vi "AlliGator Find Python Function Information.vi"(8 "error in (no error)":errorcluster, 10 "Function Menu Item Tag":string, 11 "Target":string) -> (0 "error out":errorcluster, 3 "Python Function Info":T1={"Script Path"=path "", "Function Name"="", "Function Parent Menu"="", "Function Input Parameters"=[], "Function Outputs"=[], "Function Doc String"="", "Function Display Name"="", "Function Target Type"=enum."Window Menu", "Function Target Window"="", "Parent Menu Location"="", "Item Menu Tag"="", "Is preceded by Separator"=FALSE}, 4 "Found?":bool)   [LabVIEW 2021, in "AlliGator Python Plugins.lvlib"]
doc: "Gets python function's information."
uses:
  AlliGator Python Plugins.lvlib
  AlliGator Globals, Variables & Constants.lvlib
  AlliGator Variables List.ctl
  AlliGator Python Function Information.ctl
  AlliGator Python Function List.ctl
  <vilib>/ErrorRing/Error Ring.xnode
  AlliGator Python Function Parameter Definition.ctl
  AlliGator Python Plugin Target Type.ctl
  <vilib>/Utility/error.llb/Error Cluster From Error Code.vi
  AlliGator Python Function Output Definition.ctl
panel:
  # "see the AlliGator License on the block diagram (Ctrl+E or Window:Show Block Diagram)"
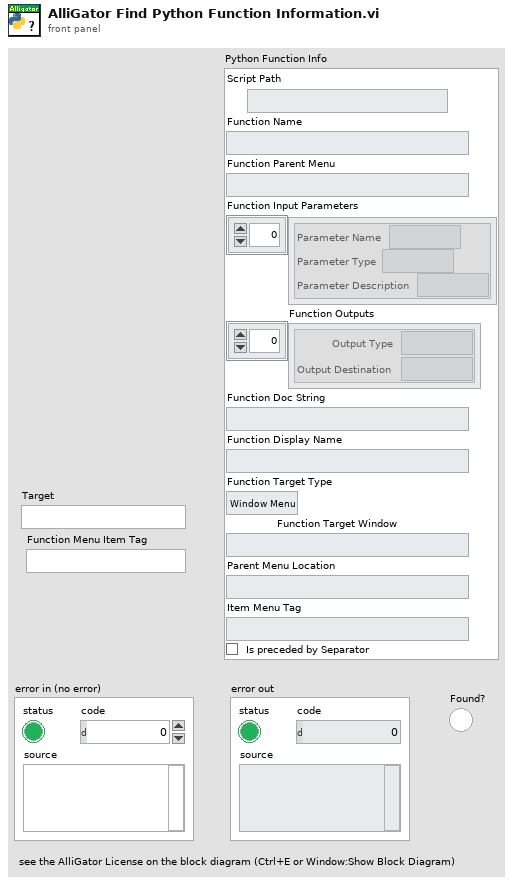
[diagram p1: front panel]
types:
  T1 = typedef "AlliGator Python Plugins.lvlib/AlliGator Python Function Information.ctl" = cluster{"Script Path":path, "Function Name":string, "Function Parent Menu":string, "Function Input Parameters":T2[], "Function Outputs":T3[], "Function Doc String":string, "Function Display Name":string, "Function Target Type":T4, "Function Target Window":string, "Parent Menu Location":string, "Item Menu Tag":string, "Is preceded by Separator":bool}
  T2 = typedef "AlliGator Python Plugins.lvlib/AlliGator Python Function Parameter Definition.ctl" = cluster{"Parameter Name":string, "Parameter Type":string, "Parameter Description":string}
  T3 = typedef "AlliGator Python Plugins.lvlib/AlliGator Python Function Output Definition.ctl" = cluster{"Output Type":string, "Output Destination":string}
  T4 = typedef "AlliGator Python Plugins.lvlib/AlliGator Python Plugin Target Type.ctl" = enum16{"Undefined", "Window Menu", "Object Menu"}
  T5 = typedef "AlliGator Python Plugins.lvlib/AlliGator Python Function List.ctl" = T1[]
  T6 = typedef "AlliGator Globals, Variables & Constants.lvlib/AlliGator Variables List.ctl" = enum16{"---- GUI ----", "GUI:Initialization Status", "GUI:State Indicators Refnum", "GUI:Original AlliGator Menu Items", "GUI:Current Action Loop State", "GUI:Script in progress", "GUI:Playback", "GUI:Loop Playback", "GUI:Search ROI Used", "GUI:Search ROI", "Decay Graph Max Legend Size", "Intensity Graph Max Legend Size", "Decay Statistics Graph Max Legend Size", "Phasor Graph Max Legend Size", "Phasor Ratio Graph Max Legend Size", "Lifetime Graph Max Legend Size", "---- Files ----", "Files:Export Dataset Frames as Individual Files", "Files:Show Batch Export Help Balloons", "Files:Frames in Dataset", "Files:ptu File Frame Start Indices", "Files:Current Frame in Dataset", "Files:Current Frame Timestamp", "Files:Dataset Loaded", "Files:Dataset Metadata", "Files:Dataset Channel", "Files:Dataset Data Description", "Files:Background Dataset Metadata", "Files:Background Dataset Channel", "Files:Background Dataset Data Description", "Files:Background File Subtraction", "Files:Background File Path", "Files:Background File Pile-up Correction", "Files:Background File Pixel Well Capacity", "Files:Background File Scaling Factor", "Files:Current Dataset Load Settings", "Files:Dataset Path", "------ Python Plugins ------", "Python Plugins:Information", "Python Plugins:Python Session", "Python Plugins:Valid Python Session?", "---- Source Image ----", "Source Image ROIs", "Current Source Image ROI", "Source Image ROI Event Refnum", "X_Source Image Display Range", "X_Source Image Palette Information", "Source Image Palette List", "Source Image Scale", "Source Image:ROI Overlay Color", "Source Image:ICCD-specific Information", "---- Image Profile Window ----", "Image Profile:Overlay ROI in Source Image", "Image Profile Window Event Refnum", "Image Profile:IntensityType", "Image Profile:Intensity Average Type", "Image Profile:Intensity-weighted SDV", "Image Profile:Box Profile Type", "Image Profile Window Open", "Image Profile:Plotted Fit Parameter", "X_Type of Displayed Image", "X_Time Gate Slider", "Source Image Overlay to Erase", "Is Displayed Image Accumulated", "White Light Image Modified", "Mask Image Modified", "Macrotime Gate Separation", "------ Phasor Graph -------", "Phasor Graph:Show Line", "---- Phasor Plot ---", "Phasor Plot Parameters Changed", "FLI Dataset Modified since last Phasor Plot Calculation", "Phasor Harmonics Data", "Selected Phasor Harmonics", "Phasor Harmonic Manager Event Refnum", "Phasor Plot ROIs", "Current Phasor Plot ROI", "Phasor Plot ROI Event Refnum", "Phasor Plot Image Reference Points", "Phasor Plot Computed", "Phasor Plot Palette Information", "Phasor Plot Palette List", "Phasor Ratio Palette Information", "Phasor Ratio Palette List", "Phasor Image Scale", "Phasor Plot Image Overlay to Erase", "Phasor Plot Image Elements to Update", "Current Phasor Plot Calculation Parameters", "Current Phasor Calibration Options", "Reset Cumulated Phasor Plot", "Phasor Ratio Reference 1", "Phasor Ratio Lifetime Reference 1", "Phasor Ratio Reference 1 Frequency", "Phasor Ratio Reference 2", "Phasor Ratio Lifetime Reference 2", "Phasor Ratio Reference 2 Frequency", "---- Decay Analysis ----", "Number of Selected Decays to Fit", "LS Fit Results", "LAR Fit Results", "BS Fit Results", "Last Decay Max - Min", "Best Fit Parameters", "Best Fit Parameter Names", "Actual Size X", "Actual Size Y", "Binning X", "Binning Y", "Actual # Gates", "Dataset Number", "Gates to...", "Gates Skipped", "Gates to keep", "Gate Step", "Gate Separation", "Reversed Gates", "Pile-up Correction", "Pixel Well Capacity", "Background Subtracted", "Background Subtraction Method", "Background Definition Range", "Background File (deprecated)", "Number of Dataset Accumulated", "Array of Accumulated Dataset Paths", "Do Averaged Datasets", "Destination File Path", "Process Plot Target", "Use 1/D as Phasor Frequency", "---- Decay Fit Parameter Map -----", "Decay Fit Parameter Map Palette Information", "Decay Fit Parameter Map Palette List", "Local Decay Graph Window Event Refnum", "------- Local Decay Window ---------", "Use normalized IRF for convolution", "----- Miscellaneous ----", "Skippable Dialog Windows Status"}
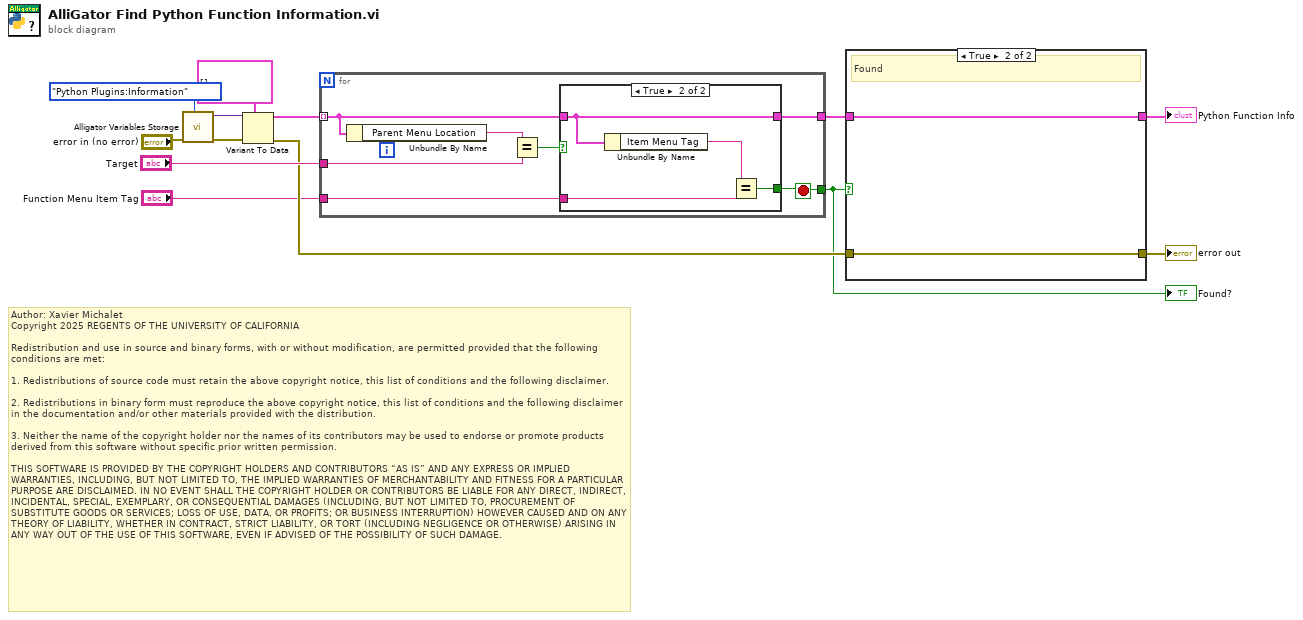
[diagram p0: block diagram]
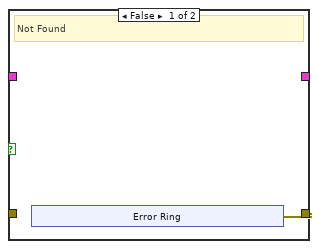
[diagram p3: hidden frame]
diagram:
  # "Author: Xavier Michalet\nCopyright 2025 REGENTS OF THE UNIVERSITY OF CALIFORNIA\n\nRedistribution and use in source and binary forms, with or without modification, are permitted provided that the following conditions are met:\n\n1. Redistributions of source code must retain the above copyright notice, this list of conditions and the following disclaimer.\n\n2. Redistributions in binary form must reproduce the above copyright notice, this list of conditions and the following disclaimer in the documentation and/or other materials provided with the distribution.\n\n3. Neither the name of the copyright holder nor the names of its contributors may be used to endorse or promote products derived from this software without specific prior written permission.\n\nTHIS SOFTWARE IS PROVIDED BY THE COPYRIGHT HOLDERS AND CONTRIBUTORS “AS IS” AND ANY EXPRESS OR IMPLIED WARRANTIES, INCLUDING, BUT NOT LIMITED TO, THE IMPLIED WARRANTIES OF MERCHANTABILITY AND FITNESS FOR A PARTICULAR PURPOSE ARE DISCLAIMED. IN NO EVENT SHALL THE COPYRIGHT HOLDER OR CONTRIBUTORS BE LIABLE FOR ANY DIRECT, INDIRECT, INCIDENTAL, SPECIAL, EXEMPLARY, OR CONSEQUENTIAL DAMAGES (INCLUDING, BUT NOT LIMITED TO, PROCUREMENT OF SUBSTITUTE GOODS OR SERVICES; LOSS OF USE, DATA, OR PROFITS; OR BUSINESS INTERRUPTION) HOWEVER CAUSED AND ON ANY THEORY OF LIABILITY, WHETHER IN CONTRACT, STRICT LIABILITY, OR TORT (INCLUDING NEGLIGENCE OR OTHERWISE) ARISING IN ANY WAY OUT OF THE USE OF THIS SOFTWARE, EVEN IF ADVISED OF THE POSSIBILITY OF SUCH DAMAGE."
  n1 = call "Alligator Variables Storage.vi"("AlliGator Variable"=AlliGator_Variables_List."Python Plugins:Information" ("Alligator Variable"), "Error In"="error in (no error)") -> ("Error Out"=w10:errorcluster, "Data out"=w11:variant)  [unwired: 7 in, 1 out]
  n2 = Variant To Data(error in=w10, type=T5 [] ("Python Function List"), Variant=w11) -> (data=w9:T5, error out=w7:errorcluster)
  n3 = for {
    tunnel: w9 -> [w15] mode=indexing
    tunnel: "Target" -> [w19]
    tunnel: "Function Menu Item Tag" -> [w17]
    tunnel: [w16] -> w1
    tunnel: [w14] -> w3
    stop <- w16 stop-if-true
    n4 = Unbundle By Name(w15) -> ("Parent Menu Location"=w20:string)
    n5 = Equal?(x=w20, y=w19) -> (x = y?=w18:bool)
    n6 = case shown="True" w18 {
      selector: w18 -> [w21 _]
      tunnel: w17 -> [_ w25]
      tunnel: [w21 w24] -> w16
      tunnel: w15 -> [_ w22]
      tunnel: [_ w22] -> w14
      frame False {
      }
      frame True {
        n7 = Unbundle By Name(w22) -> ("Item Menu Tag"=w23:string)
        n8 = Equal?(x=w23, y=w25) -> (x = y?=w24:bool)
      }
    }
  }
  "Found?" <- w1
  n9 = case shown="True" w1 {
    tunnel: w7 -> [_ w32]
    tunnel: [w26 w32] -> w6
    tunnel: w3 -> [_ w31]
    tunnel: [_ w31] -> w2
    frame False {
      # "Not Found"
      n10 = xnode "Error Ring"() -> ("error out"=w26:errorcluster)
    }
    frame True {
      # "Found"
    }
  }
  "error out" <- w6
  "Python Function Info" <- w2
